vi "SVT UFF58 Read Spectrum (Real).vi"(0 "function refnum":refnum<k20>, 11 "error in (no error)":errorcluster) -> (3 "ID lines (1-3)":T2, 4 "dup function refnum":refnum<k20>, 6 "spectrum":T1(graph), 15 "error out":errorcluster)   [LabVIEW 2017, in "SoundVib_UFF58.lvlib"]
doc: "Reads data from a UFF58 (universal file format) function specified by the <B>function refnum</B> input. This VI also reads the fields in records 1, 2, and 3, returned by ID lines (1-3). You can read a single time domain waveform, a single frequency spectrum, the real and imaginary parts of a frequency spectrum, and any data from a function. The default instance, SVT UFF58 Read Time Waveform, reads a single time domain waveform from a function specified by the <B>function refnum</B> input. Wire data to the <B>function refnum</B> input to determine the polymorphic instance to use or manually select the instance."
uses:
  <vilib>/addons/Sound and Vibration/svt_UFF58/SoundVib_UFF58.lvlib
  <vilib>/addons/Sound and Vibration/svt_UFF58/subVIs/sv_IDLines123.ctl
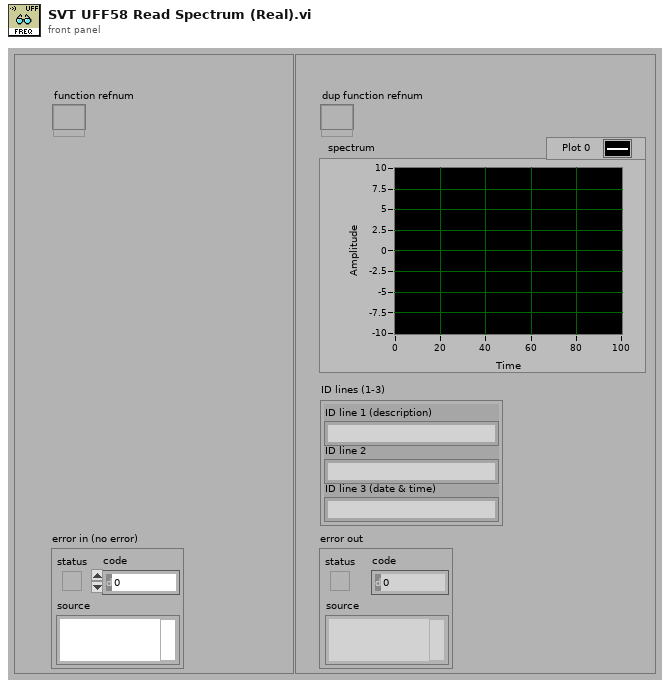
[diagram p1: front panel]
types:
  T1 = cluster{"abscissa minimum":dbl, "abscissa increment":dbl, "data":dbl[]}
  T2 = typedef "SoundVib_UFF58.lvlib/sv_IDLines123.ctl" = cluster{"ID line 1 (description)":string, "ID line 2":string, "ID line 3 (date & time)":string}
  T3 = typedef "SoundVib_UFF58.lvlib/sv_UFF58 DOF.ctl" = cluster{"function type":T4, "function ID number":i32, "version number":i32, "load case ID number":i32, "response entity name":string, "response node":i32, "response direction":T5, "reference entity name":string, "reference node":i32, "reference direction":T5}
  T4 = typedef "SoundVib_UFF58.lvlib/sv_FunctionType.ctl" = enum16{"general or unknown", "time response", "auto spectrum", "cross spectrum", "frequency response function", "transmissibility", "coherence", "auto correlation", "cross correlation", "power spectral density (PSD)", "energy spectral density (ESD)", "probability density function", "spectrum", "cumulative frequency distribution", "peaks valley", "stress/cycles", "strain/cycles", "orbit", "mode indicator function", "force pattern", "partial power", "partial coherence", "eigenvalue", "eigenvector", "shock response spectrum", "finite impulse response filter", "multiple coherence", "order function", "phase compensation"}
  T5 = typedef "SoundVib_UFF58.lvlib/sv_UFF58 Response Direction.ctl" = i32
  T6 = typedef "SoundVib_UFF58.lvlib/sv_UFF58 Data Form.ctl" = cluster{"ordinate data type":u16, "number of data values/pairs":i32, "abscissa spacing":enum16{"uneven", "even"}, "abscissa minimum":dbl, "abscissa increment":dbl}
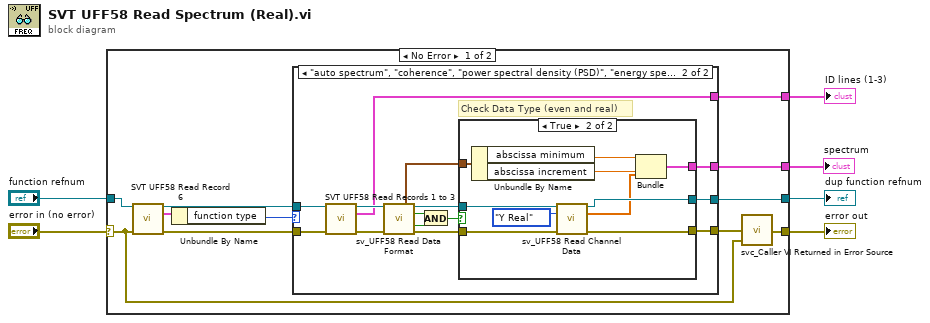
[diagram p0: block diagram]
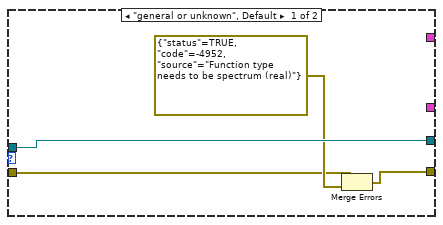
[diagram p2: hidden frame]
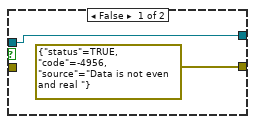
[diagram p3: hidden frame]
diagram:
  n1 = case shown="No Error" "error in (no error)" {
    selector: "error in (no error)" -> [w9 w48]
    tunnel: [w13 w49] -> w1
    tunnel: [w16 w48] -> w6
    tunnel: "function refnum" -> [w11 w49]
    tunnel: [w14 _] -> w5
    tunnel: [w17 _] -> w3
    frame No Error {
      n2 = call <vilib>:"SVT UFF58 Read Record 6.vi"("function refnum"=w11, "error in (no error)"=w9) -> ("dup function refnum"=w8:refnum<k20>, "DOF identification"=w12:T3, "error out"=w10:errorcluster)  [unwired: 11 in]
      n3 = Unbundle By Name(w12) -> ("function type"=w7:T4)
      n4 = case shown="\"auto spectrum\", \"coherence\", \"power spectral density (PSD)\", \"energy spectral density (ESD)\", \"spectrum\", \"partial power\", \"partial coherence\", \"shock response spectrum\"" w7 {
        tunnel: [_ w33] -> w17
        tunnel: [w18 w31] -> w15
        tunnel: [_ w29] -> w14
        tunnel: [w21 w24] -> w13
        tunnel: w10 -> [w19 w23]
        tunnel: w8 -> [w21 w22]
        frame "general or unknown", Default {
          n5 = Merge Errors(w19, errorcluster {"status"=TRUE, "code"=-4952, "source"="Function type needs to be spectrum (real)"} ("error out")) -> (w18:errorcluster)
        }
        frame "auto spectrum", "coherence", "power spectral density (PSD)", "energy spectral density (ESD)", "spectrum", "partial power", "partial coherence", "shock response spectrum" {
          # "Check Data Type (even and real)"
          n6 = call <vilib>:"SVT UFF58 Read Records 1 to 3.vi"("function refnum"=w22, "error in (no error)"=w23) -> ("dup function refnum"=w35:refnum<k20>, "ID lines (1-3)"=w33:T2, "error out"=w34:errorcluster)  [unwired: 11 in]
          n7 = call <vilib>:"sv_UFF58 Read Data Format.vi"("function refnum"=w35, "error in (no error)"=w34) -> ("data form"=w30:T6, "dup function refnum"=w28:refnum<k20>, "even"=w26:bool, "real"=w27:bool, "error out"=w32:errorcluster)  [unwired: 9 in]
          n8 = And(x=w26, y=w27) -> (x .and. y?=w25:bool)
          n9 = case shown="True" w25 {
            tunnel: w28 -> [w37 w44]
            tunnel: w32 -> [_ w43]
            tunnel: [w37 w46] -> w24
            tunnel: [errorcluster {"status"=TRUE, "code"=-4956, "source"="Data is not even and real "} ("error out") w45] -> w31
            tunnel: [_ w41] -> w29
            tunnel: w30 -> [_ w42]
            frame False {
            }
            frame True {
              n10 = Unbundle By Name(w42) -> ("abscissa minimum"=w38:dbl, "abscissa increment"=w39:dbl)
              n11 = call <vilib>:"sv_UFF58 Read Channel Data.vi"("function refnum"=w44, "channel to read"=enum16{"X", "Y Real", "Y Imaginary"}."Y Real" ("data to read"), "error in (no error)"=w43) -> ("dup function refnum"=w46:refnum<k20>, "data"=w40:dbl[], "error out"=w45:errorcluster)  [unwired: 10 in]
              n12 = Bundle("abscissa minimum"=w38, "abscissa increment"=w39, "data"=w40) -> (w41:T1)  [unwired: 1 in]
            }
          }
        }
      }
      n13 = call <vilib>:"svc_Caller VI Returned in Error Source.vi"("warning input to caller"=w9, "error in (no error)"=w15) -> ("error out"=w16:errorcluster)  [unwired: 3 in]
    }
    frame Error {
    }
  }
  "error out" <- w6
  "spectrum" <- w5
  "ID lines (1-3)" <- w3
  "dup function refnum" <- w1
